vi "Is ProjectItem Virtual Folder.vi"(8 "Error In":errorcluster, 11 "ProjectItem Refnum":refnum<vi>) -> (0 "Error Out":errorcluster, 3 "Is Virtual Folder?":bool)   [LabVIEW 2022 SP3]
doc: "This VI outputs True if and only if the input Project Item is a Virtual Folder (as opposed to an auto-populating folder).\n\nPlease note that an auto-populating folder and a virtual folder have the same Type \"{D60740D6-F254-4BBC-5675-8858F35B820E}\" and TypeString: \"Folder\".\n\nHowever, the \"Auto-Populating Path\" property can be used to distinguish between the two. That property returns <Not A Path> for a virtual folder, and returns a valid path for an auto-populating folder."
panel:
  # "Development\nControls or indicators that are useful for development or testing, but which are not outputs of the VI."
  # "Input\nInputs to the VI"
  # "Output\nOutputs of the VI"
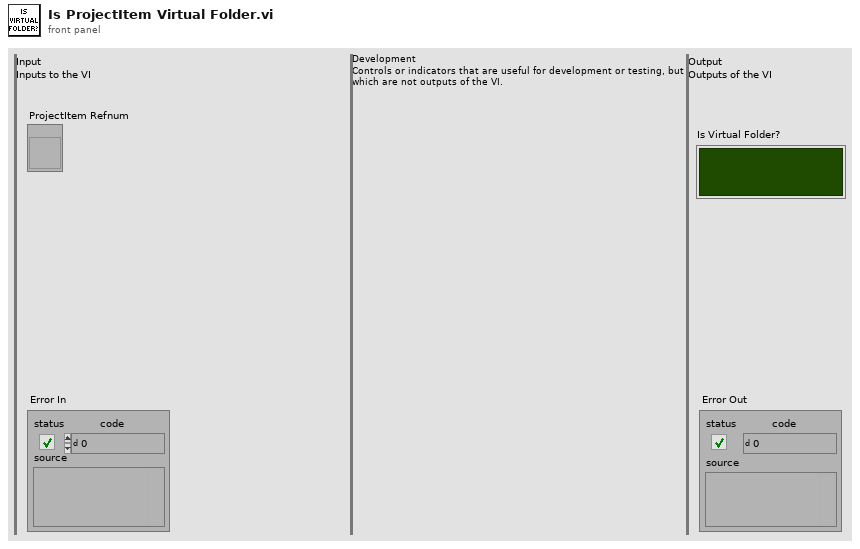
[diagram p1: front panel]
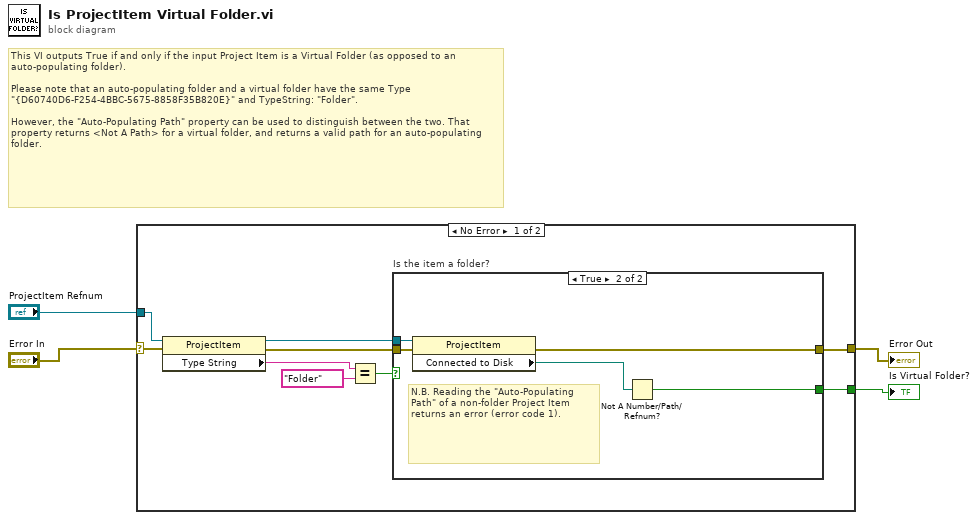
[diagram p0: block diagram]
diagram:
  # "This VI outputs True if and only if the input Project Item is a Virtual Folder (as opposed to an auto-populating folder).\n\nPlease note that an auto-populating folder and a virtual folder have the same Type \"{D60740D6-F254-4BBC-5675-8858F35B820E}\" and TypeString: \"Folder\".\n\nHowever, the \"Auto-Populating Path\" property can be used to distinguish between the two. That property returns <Not A Path> for a virtual folder, and returns a valid path for an auto-populating folder."
  n1 = case shown="No Error" "Error In" {
    selector: "Error In" -> [w13 w20]
    tunnel: [w6 w20] -> w3
    tunnel: "ProjectItem Refnum" -> [w12 _]
    tunnel: [w5 _] -> w1
    frame No Error {
      n2 = property class="ProjectItem"(reference=w12, error in=w13) -> (reference out=w8:refnum<vi>, error out=w9:errorcluster, "Type String"=w11:string)
      n3 = Equal?(x=w11, y="Folder") -> (x = y?=w7:bool)
      n4 = case "Is the item a folder?" shown="True" w7 {
        tunnel: w9 -> [w14 w19]
        tunnel: w8 -> [_ w18]
        tunnel: [w14 w17] -> w6
        tunnel: [_ w15] -> w5
        frame False {
        }
        frame True {
          # "N.B. Reading the \"Auto-Populating Path\" of a non-folder Project Item returns an error (error code 1)."
          n5 = property class="ProjectItem"(reference=w18, error in=w19) -> (error out=w17:errorcluster, "Connected to Disk"=w16:path)  [unwired: 1 out]
          n6 = Not A Number/Path/Refnum?(number/path/refnum=w16) -> (NaN/Path/Refnum?=w15:bool)
        }
      }
    }
    frame Error {
    }
  }
  "Error Out" <- w3
  "Is Virtual Folder?" <- w1
